vi "Sequencer Main.vi"() -> ()   [LabVIEW 2022 SP3]
uses:
  Sequencer State.ctl
  Controls/All Loop Status.ctl
  Sub VI's/Global 1.vi
  <vilib>/Utility/file.llb/Write Delimited Spreadsheet (string).vi
panel:
  out "Sync":bool
  in  "Launch Time":timestamp format="%<%x %.3X>T"
  in  "Ready Seq":bool
  in  "Load Seq":bool
  in  "Stop Sequence":bool
  in  "Update Seq":bool
  in  "Select Sequencer File*":path
  out "Instrumentaion Test Bench Count Down Timer":dbl
  in  "Abort Sequence":bool
  out "SEQ HL":bool
  out "DO HL":bool
  out "AO HL":bool
  in  "Tab Control":T1(tab)
  out "Display":string[][](table)
  in  "Edit data":string[][](table)
  in  "Save Changes":bool
  out "Feed":string
  out "AO State":cluster{"DO":dbl, "CN":string}[](array[cluster])
  out "DO State":cluster{"DO":bool, "CN":string}[](array[cluster])
  # "ITB SEQUENCER"
  # "Agnikul Cosmos Private Limited"
  # "Access:Read Only"
  # "Access:Read/Write"
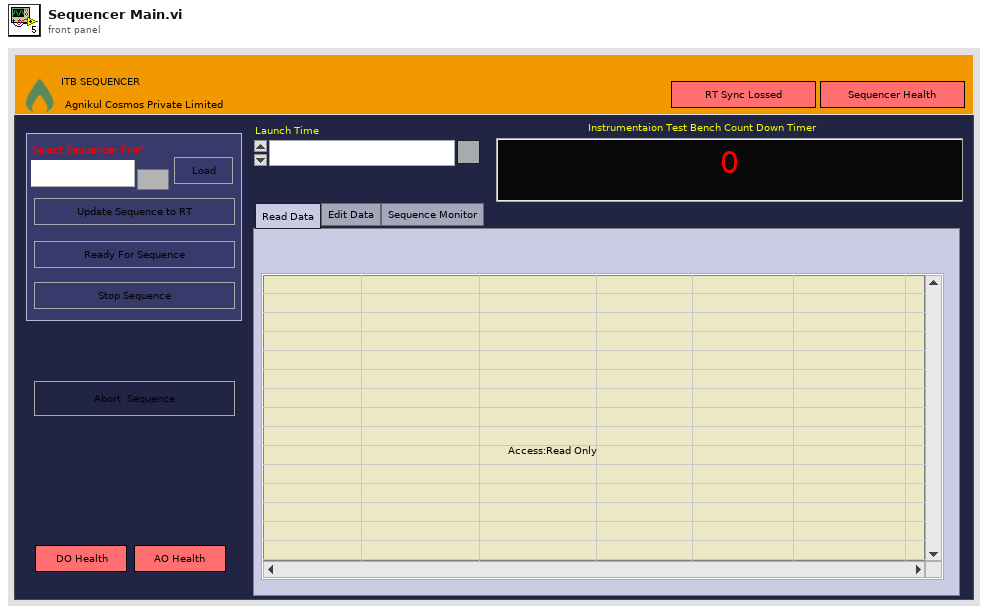
[diagram p1: front panel]
types:
  T1 = enum32{"Read Data", "Edit Data", "Sequence Monitor"}
  T2 = cluster{"Select Sequencer File*":path, "DO":cluster{"CDT":dbl, "Position":bool, "Component ID":string}[], "AO":cluster{"CDT":dbl, "Range":dbl, "Component ID":string}[], "Launch Time":timestamp}
  T3 = typedef "Sequencer State.ctl" = enum16{"Initialize", "Polevent", "Read file", "Update Seq", "Write AO", "Write DO", "Exit"}
  T4 = enum16{"Init", "Read 'All'", "Read 'n'", "Read '1'", "Write '1'", "Write 'n'", "Write 'All'"}
  T5 = cluster{"AO":cluster{"CDT":dbl, "Range":dbl, "Component ID":string}[], "DO":cluster{"CDT":dbl, "Position":bool, "Component ID":string}[], "Launch Time":timestamp}
  T6 = typedef "All Loop Status.ctl" = enum16{"AI", "AO", "DI", "DO", "TC", "Strain", "ACC", "RT", "Log", "Seq", "Sync"}
  T7 = cluster{"CDT":dbl, "Range":dbl, "Component ID":string}[]
  T8 = cluster{"CDT":dbl, "Position":bool, "Component ID":string}[]
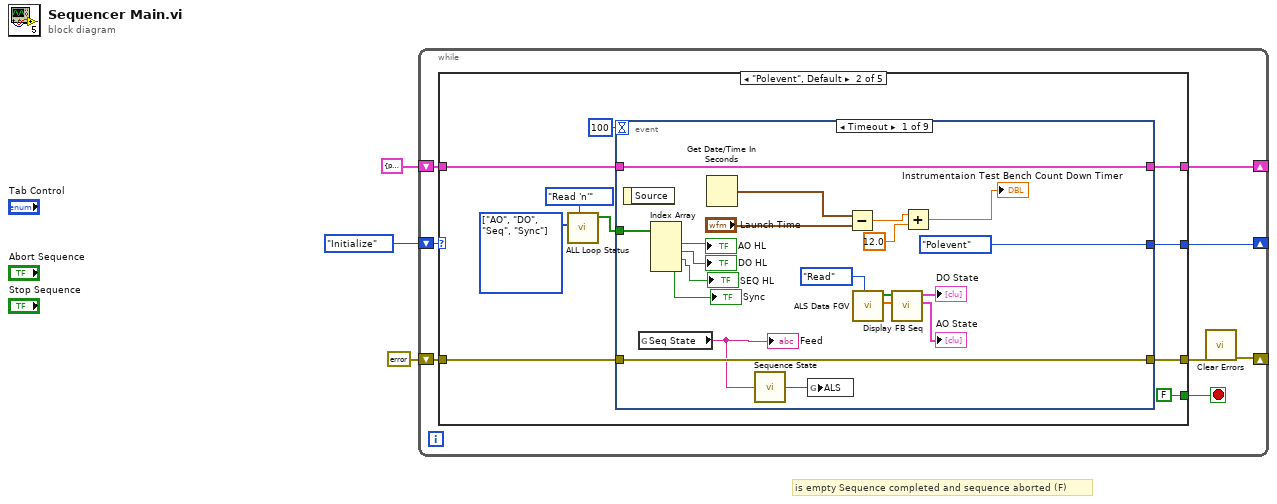
[diagram p0: block diagram]
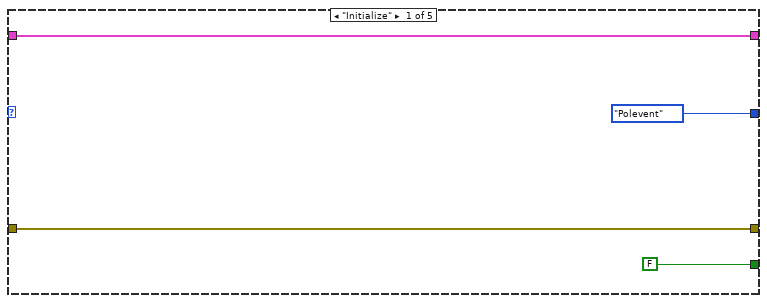
[diagram p2: hidden frame]
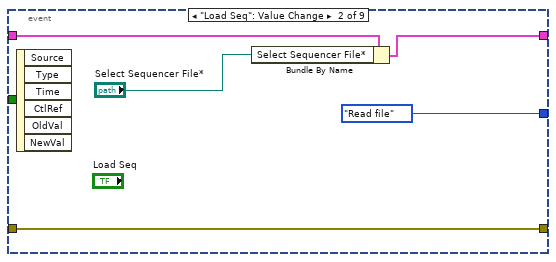
[diagram p3: hidden frame]
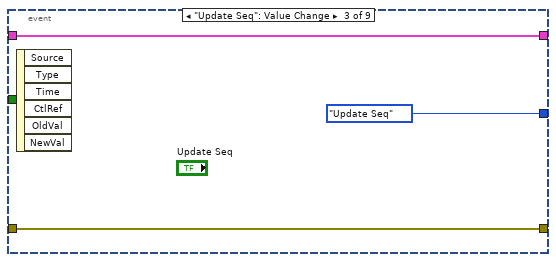
[diagram p4: hidden frame]
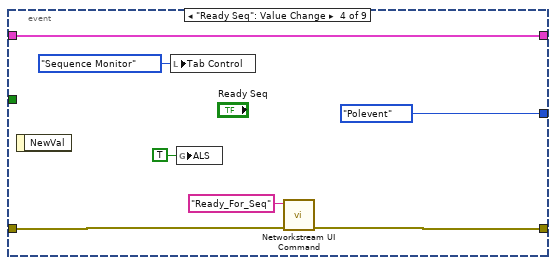
[diagram p5: hidden frame]
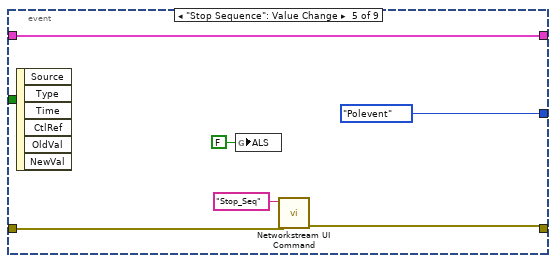
[diagram p6: hidden frame]
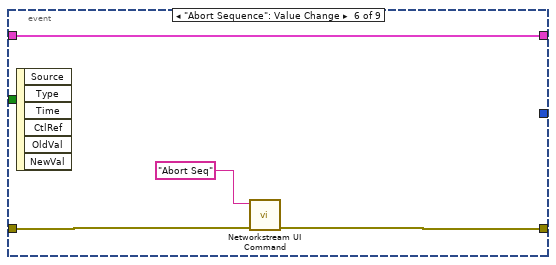
[diagram p7: hidden frame]
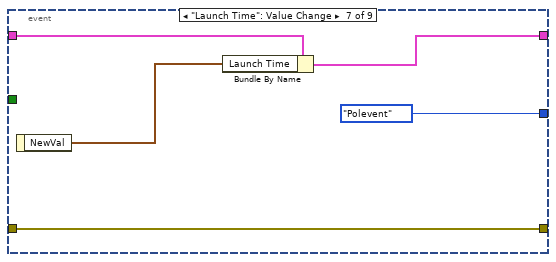
[diagram p8: hidden frame]
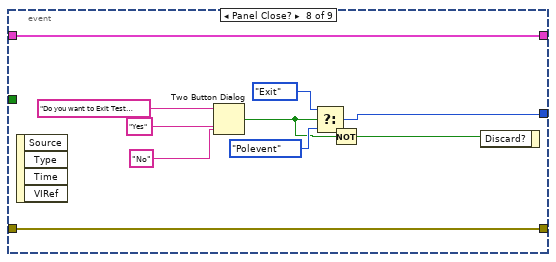
[diagram p9: hidden frame]
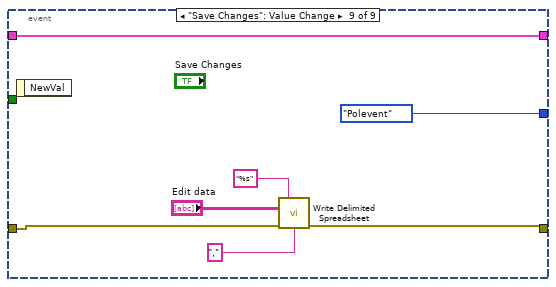
[diagram p10: hidden frame]
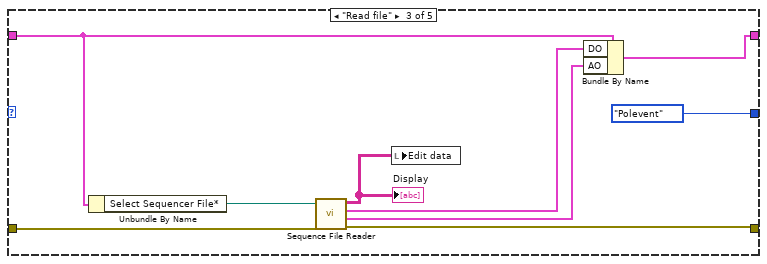
[diagram p11: hidden frame]
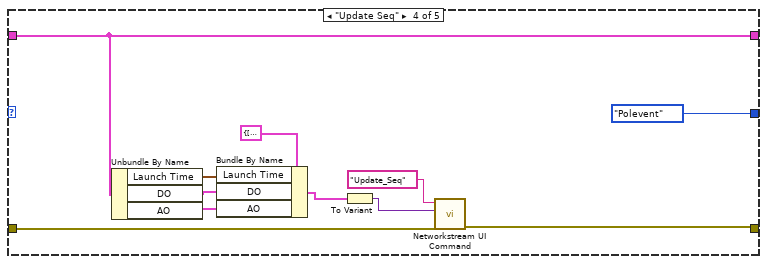
[diagram p12: hidden frame]
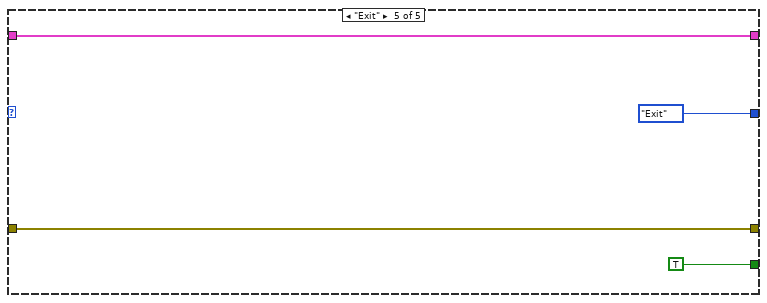
[diagram p13: hidden frame]
diagram:
  # "is empty Sequence completed and sequence aborted (F)"
  n1 = while {
    shift-right: [w10] -> _
    shift-left: Sequencer_State."Initialize" ("Enum") -> [w11]
    shift-right: [w7] -> _
    shift-left: T2 {"Select Sequencer File*"=path "", "DO"=[], "AO"=[], "Launch Time"=timestamp(0 s since 1904-01-01)} -> [w8]
    shift-right: [w4] -> _
    shift-left: errorcluster {"status"=FALSE, "code"=0, "source"=""} ("error constant") -> [w6]
    stop <- w9 stop-if-true
    n2 = case shown="\"Polevent\", Default" w11 {
      tunnel: [Sequencer_State."Polevent" ("Enum") w25 Sequencer_State."Polevent" ("Enum") Sequencer_State."Polevent" ("Enum") Sequencer_State."Exit" ("Enum")] -> w10
      tunnel: [FALSE FALSE _ _ TRUE] -> w9
      tunnel: w8 -> [w13 w23 w96 w108 w114]
      tunnel: [w13 w22 w97 w108 w114] -> w7
      tunnel: w6 -> [w12 w20 w100 w111 w113]
      tunnel: [w12 w19 w99 w110 w113] -> w5
      frame "Initialize" {
      }
      frame "Polevent", Default {
        w17 = T6[] [enum."AO", enum."DO", enum."Seq", enum."Sync"] items=["AI", "AO", "DI", "DO", "TC", "Strain", "ACC", "RT", "Log", "Seq", "Sync"] ("Loops")
        n3 = call "ALL Loop Status.vi"("Option"=T4."Read 'n'", "Loops"=w17) -> ("Status List Out"=w16:bool[])  [unwired: 7 in, 2 out]
        n4 = event shown="[0] Timeout" {
          selector: _ -> [_ _ _ _ _ _ _ _ _]
          dyn-events: _ -> [_ _ _ _ _ _ _ _ _]
          timeout: 100 -> [_ _ _ _ _ _ _ _ _]
          tunnel: [Sequencer_State."Polevent" ("Enum") Sequencer_State."Read file" ("Enum") Sequencer_State."Update Seq" ("Enum") Sequencer_State."Polevent" ("Enum") Sequencer_State."Polevent" ("Enum") _ Sequencer_State."Polevent" ("Enum") w78 Sequencer_State."Polevent" ("Enum")] -> w25
          tunnel: w23 -> [w43 w50 w53 w60 w66 w70 w73 w85 w92]
          tunnel: [w43 w49 w53 w60 w66 w70 w74 w85 w92] -> w22
          tunnel: w20 -> [w44 w46 w52 w59 w63 w68 w75 w84 w89]
          tunnel: [w44 w46 w52 w58 w62 w67 w75 w84 w88] -> w19
          tunnel: w16 -> [w35 _ _ _ _ _ _ _ _]
          event Timeout {
            n5 = event-data() -> ()  [unwired: 1 in, 1 out]
            n6 = global read "Global 1.vi" "Seq State"() -> (w31:string)
            "Feed" <- w31
            n7 = Index Array(array=w35) -> (element #1=→"AO HL":bool, element #2=→"DO HL":bool, element #3=→"SEQ HL":bool, element #4=→"Sync":bool)  [unwired: 4 in]
            n8 = Get Date/Time In Seconds() -> (seconds since 1Jan1904=w42:timestamp)
            n9 = call "Sequence State.vi"("y"=w31) -> ("result"=w30:bool)  [unwired: 4 in]
            n10 = global write "Global 1.vi" "ALS"(w30) -> ()
            n11 = Subtract(x=w42, y="Launch Time") -> (x-y=w28:dbl)
            n12 = call "ALS Data FGV.vi"("Enum"=enum16{"Read", "Write"}."Read") -> ("ALS AO out"=w38:dbl[], "ALS DO out"=w37:bool[])  [unwired: 8 in, 1 out]
            n13 = call "Display FB Seq.vi"("ALS AO in"=w38, "ALS DO in"=w37) -> ("AO State"=→"AO State":cluster{"DO":dbl, "CN":string}[], "DO State"=→"DO State":cluster{"DO":bool, "CN":string}[])  [unwired: 8 in]
            n14 = Add(x=w28, y=12.0) -> (x+y=→"Instrumentaion Test Bench Count Down Timer":dbl)
          }
          event "Load Seq": Value Change {
            n15 = event-data() -> ()  [unwired: 1 in, 6 out]
            n16 = Bundle By Name(cluster=w50, "Select Sequencer File*"="Select Sequencer File*") -> (w49:T2)
          }
          event "Update Seq": Value Change {
            n17 = event-data() -> ()  [unwired: 1 in, 6 out]
          }
          event "Ready Seq": Value Change {
            n18 = event-data() -> ()  [unwired: 1 in, 1 out]
            n19 = local write "Tab Control"(T1."Sequence Monitor" ("Tab Control")) -> ()
            n20 = global write "Global 1.vi" "ALS"(TRUE ("ALS")) -> ()
            n21 = call "Networkstream UI Command.vi"("error in"=w59, "Message"="Ready_For_Seq") -> ("error out"=w58:errorcluster)  [unwired: 9 in]
          }
          event "Stop Sequence": Value Change {
            n22 = event-data() -> ()  [unwired: 1 in, 6 out]
            n23 = global write "Global 1.vi" "ALS"(FALSE ("ALS")) -> ()
            n24 = call "Networkstream UI Command.vi"("error in"=w63, "Message"="Stop_Seq") -> ("error out"=w62:errorcluster)  [unwired: 9 in]
          }
          event "Abort Sequence": Value Change {
            n25 = event-data() -> ()  [unwired: 1 in, 6 out]
            n26 = call "Networkstream UI Command.vi"("error in"=w68, "Message"="Abort Seq") -> ("error out"=w67:errorcluster)  [unwired: 9 in]
          }
          event "Launch Time": Value Change {
            n27 = event-data() -> ("NewVal"=w71:timestamp)  [unwired: 1 in]
            n28 = Bundle By Name(cluster=w73, "Launch Time"=w71) -> (w74:T2)
          }
          event Panel Close? {
            n29 = event-data() -> ()  [unwired: 1 in, 4 out]
            n30 = Two Button Dialog(message="Do you want to Exit Test Bench?", 1:"No" ("F button name (\"Cancel\")"), 2:"Yes" ("T button name (\"OK\")")) -> (T button?=w77:bool)
            n31 = Select(t=Sequencer_State."Exit" ("Enum"), s=w77, f=Sequencer_State."Polevent" ("Enum")) -> (s? t:f=w78:T3)
            n32 = Not(x=w77) -> (.not. x?=w76:bool)
            n33 = event-data("Discard?"=w76) -> ()  [unwired: 1 in, 1 out]
          }
          event "Save Changes": Value Change {
            n34 = event-data() -> ()  [unwired: 1 in, 1 out]
            n35 = call-poly <vilib>:"Write Delimited Spreadsheet.vi"("format (%s)"="%s", "2D data"="Edit data", "error in (no error)"=w89, "delimiter (\\t)"="," ("delimiter (\\t)")) -> ("error out"=w88:errorcluster)  [unwired: 10 in, 1 out]
          }
        }
      }
      frame "Read file" {
        n36 = Unbundle By Name(w96) -> ("Select Sequencer File*"=w98:path)
        n37 = call "Sequence File Reader.vi"("error in"=w100, "Select Sequencer File*"=w98) -> ("error out"=w99:errorcluster, "AO"=w94:T7, "DO"=w95:T8, "all rows"=w93:string[][])  [unwired: 6 in]
        "Display" <- w93
        n38 = local write "Edit data"(w93) -> ()
        n39 = Bundle By Name(cluster=w96, "DO"=w95, "AO"=w94) -> (w97:T2)
      }
      frame "Update Seq" {
        n40 = Unbundle By Name(w108) -> ("Launch Time"=w102:timestamp, "DO"=w106:T8, "AO"=w105:T7)
        n41 = Bundle By Name(cluster=T5 {"AO"=[], "DO"=[], "Launch Time"=timestamp(0 s since 1904-01-01)}, "Launch Time"=w102, "DO"=w106, "AO"=w105) -> (w104:T5)
        n42 = To Variant(anything=w104) -> (Variant=w103:variant)
        n43 = call "Networkstream UI Command.vi"("error in"=w111, "Data"=w103, "Message"="Update_Seq") -> ("error out"=w110:errorcluster)  [unwired: 8 in]
      }
      frame "Exit" {
      }
    }
    n44 = call <vilib>:"Clear Errors.vi"("error in (no error)"=w5) -> ("error out"=w4:errorcluster)  [unwired: 5 in, 1 out]
  }
